vi "Load Program Process AHUold.vi"(0 "Enable":bool=TRUE, 5 "error in (no error)":errorcluster) -> (1 "Speed Command Test":bool, 2 "Temperature Sensor Calibration Test":bool, 3 "Burn-in Test":bool, 4 "Automation":bool, 6 "Performance Test":bool, 7 "Enable Test":bool, 8 "Communication Test":bool, 9 "Sealing Test":bool, 10 "CANBus Resistance Test":bool, 11 "Bonding Resistance":bool, 12 "Insulation Resistance Test":bool, 13 "Functional Test Procedure":bool, 14 "Power Supply Voltages":bool, 15 "Power Supply Testing":bool, 16 "Manufacturing Defects":bool, 17 "Visual Inspection":bool, 18 "OK":bool, 19 "error out":errorcluster)   [LabVIEW 2017]
doc: "Displays a standard dialog box that prompts users to enter information, such as a user name and password.\n--------------------\n\nThis Express VI is configured as follows:\n\nMessage to Display to the User:Please select the test(s) you want to execute(s).\nThe inputs are: \nCheckbox: Visual Inspection\nCheckbox: Manufacturing Defects\nCheckbox: Power Supply Testing\nCheckbox: Power Supply Voltages\nCheckbox: Functional Test Procedure\nCheckbox: Insulation Resistance Test\nCheckbox: Bonding Resistance\nCheckbox: CANBus Resistance Test\nCheckbox: Sealing Test\nCheckbox: Communication Test"
panel:
  in  "Burn-in Test":bool
  in  "Temperature Sensor Calibration Test":bool
  in  "Speed Command Test":bool
  in  "Enable Test":bool
  in  "Performance Test":bool
  in  "Communication Test":bool
  in  "Sealing Test":bool
  in  "CANBus Resistance Test":bool
  in  "Bonding Resistance":bool
  in  "Insulation Resistance Test":bool
  in  "Functional Test Procedure":bool
  in  "Power Supply Voltages":bool
  in  "Power Supply Testing":bool
  in  "Manufacturing Defects":bool
  in  "Visual Inspection":bool
  out "String":string="Please select the test(s) you want to execute(s)."
  in  "Cancel":bool
  in  "OK2":bool
  in  "Automation":bool caption="OK1"
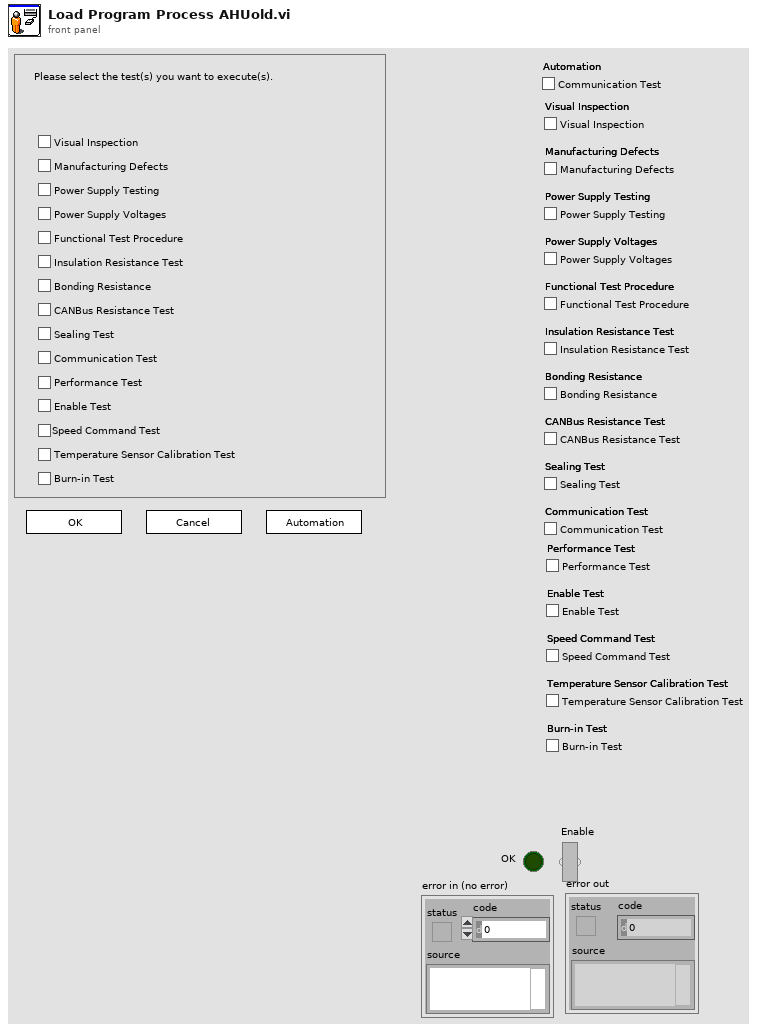
[diagram p1: front panel]
types:
  T1 = cluster{"Input Name":string, "Input Data Type":i32}[]
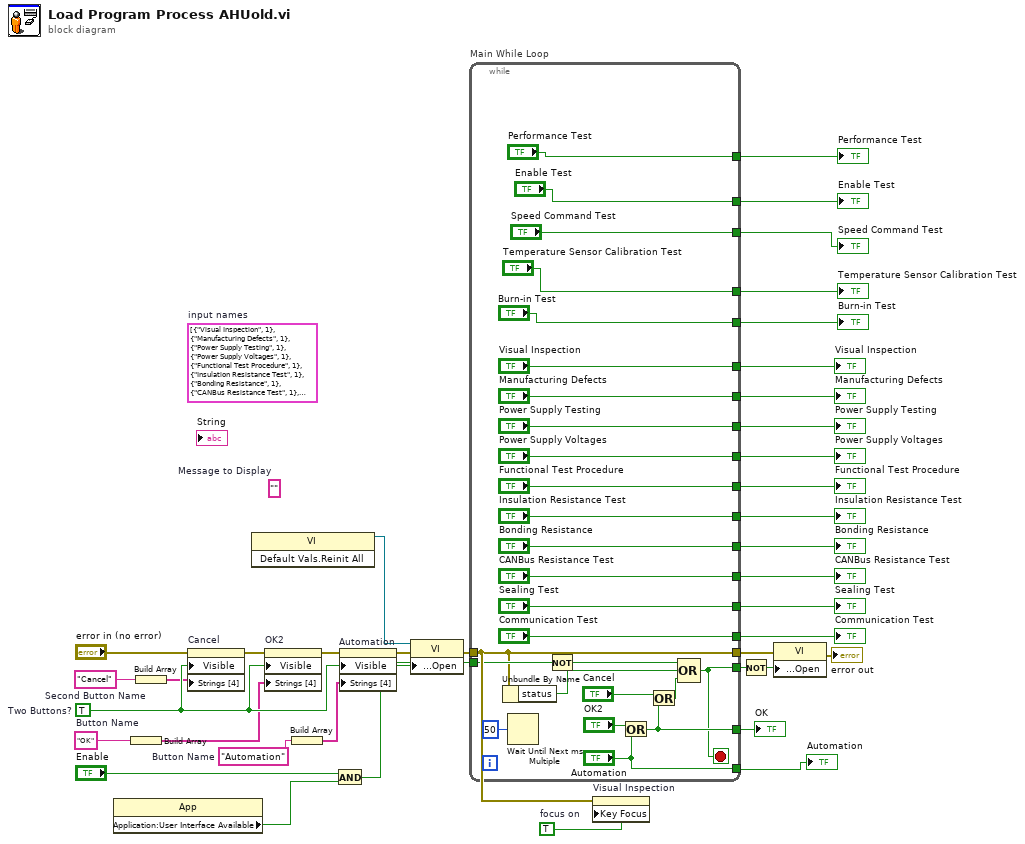
[diagram p0: block diagram]
diagram:
  w2 = "Automation"  # Button Name
  w18 = TRUE  # focus on
  (unwired) T1 [{"Input Name"="Visual Inspection", "Input Data Type"=1}, {"Input Name"="Manufacturing Defects", "Input Data Type"=1}, {"Input Name"="Power Supply Testing", "Input Data Type"=1}, {"Input Name"="Power Supply Voltages", "Input Data Type"=1}, {"Input Name"="Functional Test Procedure", "Input Data Type"=1}, {"Input Name"="Insulation Resistance Test", "Input Data Type"=1}, {"Input Name"="Bonding Resistance", "Input Data Type"=1}, {"Input Name"="CANBus Resistance Test", "Input Data Type"=1}, {"Input Name"="Sealing Test", "Input Data Type"=1}, {"Input Name"="Communication Test", "Input Data Type"=1}]  # input names
  w31 = "Cancel"  # Second Button Name
  w29 = "OK"  # Button Name
  (unwired) ""  # Message to Display
  w38 = TRUE  # Two Buttons?
  n1 = property class="App"() -> ("Application:User Interface Available"=w21:bool)  [unwired: 2 in, 2 out]
  n2 = Build Array(w29) -> (w30:string[])
  n3 = Build Array(w31) -> (w32:string[])
  n4 = property on="Cancel" class="Bool"(error in="error in (no error)", "Visible"=w38, "Strings [4]"=w32) -> (error out=w36:errorcluster)  [unwired: 1 in, 1 out]
  n5 = invoke class="VI" method="Default Vals.Reinit All"() -> (reference out=w20:refnum<vi>)  [unwired: 3 in, 2 out]
  n6 = property on="OK2" class="Bool"(error in=w36, "Visible"=w38, "Strings [4]"=w30) -> (error out=w35:errorcluster)  [unwired: 1 in, 1 out]
  n7 = Build Array(w2) -> (w3:string[])
  n8 = And(x="Enable", y=w21) -> (x .and. y?=w22:bool)
  n9 = property on="Automation" class="Bool"(error in=w35, "Visible"=w38, "Strings [4]"=w3) -> (error out=w28:errorcluster)  [unwired: 1 in, 1 out]
  n10 = property class="VI"(reference=w20, error in=w28, "Front Panel Window:Open"=w22) -> (error out=w27:errorcluster)  [unwired: 1 out]
  n11 = while "Main While Loop" {
    tunnel: [w61] -> w37
    tunnel: w22 -> [w60]
    tunnel: [w58] -> w33
    tunnel: w27 -> [w57]
    tunnel: [w57] -> w25
    tunnel: ["Visual Inspection"] -> w19
    tunnel: ["Manufacturing Defects"] -> w17
    tunnel: ["Power Supply Testing"] -> w16
    tunnel: ["Power Supply Voltages"] -> w15
    tunnel: ["Functional Test Procedure"] -> w14
    tunnel: ["Insulation Resistance Test"] -> w13
    tunnel: ["Bonding Resistance"] -> w12
    tunnel: ["CANBus Resistance Test"] -> w11
    tunnel: ["Sealing Test"] -> w10
    tunnel: ["Communication Test"] -> w9
    tunnel: ["Performance Test"] -> w8
    tunnel: ["Enable Test"] -> w7
    tunnel: ["Speed Command Test"] -> w6
    tunnel: ["Temperature Sensor Calibration Test"] -> w5
    tunnel: ["Burn-in Test"] -> w4
    tunnel: ["Automation"] -> w1
    stop <- w58 stop-if-true
    n12 = Unbundle By Name(w57) -> ("status"=w55:bool)
    n13 = Wait Until Next ms Multiple(millisecond multiple=u32 50) -> ()  [unwired: 1 out]
    n14 = Not(x=w60) -> (.not. x?=w59:bool)
    n15 = Or(x="OK2", y="Automation") -> (x .or. y?=w61:bool)
    n16 = Or(x="Cancel", y=w61) -> (x .or. y?=w56:bool)
    n17 = Compound Arithmetic op=OR(w59, w55, w56) -> (w58:bool)
  }
  "OK" <- w37
  "Visual Inspection" <- w19
  "Manufacturing Defects" <- w17
  "Power Supply Testing" <- w16
  "Power Supply Voltages" <- w15
  "Functional Test Procedure" <- w14
  "Insulation Resistance Test" <- w13
  "Bonding Resistance" <- w12
  "CANBus Resistance Test" <- w11
  "Sealing Test" <- w10
  "Communication Test" <- w9
  "Performance Test" <- w8
  "Enable Test" <- w7
  "Speed Command Test" <- w6
  "Temperature Sensor Calibration Test" <- w5
  "Burn-in Test" <- w4
  "Automation" <- w1
  n18 = property on="Visual Inspection" class="Bool (strict)"(error in=w27, "Key Focus"=w18) -> ()  [unwired: 1 in, 2 out]
  n19 = Not(x=w33) -> (.not. x?=w34:bool)
  n20 = property class="VI"(error in=w25, "Front Panel Window:Open"=w34) -> (error out=→"error out":errorcluster)  [unwired: 1 in, 1 out]
